vi "Compare VIs.vi"(7 "Interactive? (F)":bool, 8 "error in (no error)":errorcluster, 9 "VI Comparison Options":T1={"VI Attributes?"=TRUE, "Front Panel"=FALSE, "Front Panel Position/Size"=FALSE, "Block Diagram"=TRUE, "Block Diagram Cosmetic"=FALSE, "Block Diagram Position/Size"=FALSE}, 10 "VI Path 2":path, 11 "VI Path 1":path) -> (0 "error out":errorcluster, 3 "Different?":bool)   [LabVIEW 2016, in "SLL Scripting.lvlib"]
doc: "Compare two VIs provided their path."
uses:
  SLL Scripting.lvlib
  _Typedefs/VI Comparison Options.ctl
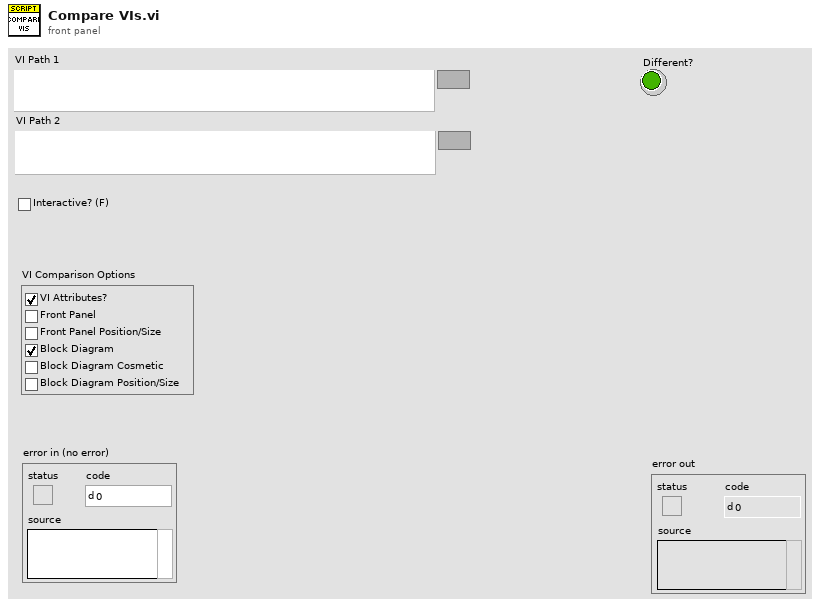
[diagram p1: front panel]
types:
  T1 = typedef "SLL Scripting.lvlib/VI Comparison Options.ctl" = cluster{"VI Attributes?":bool, "Front Panel":bool, "Front Panel Position/Size":bool, "Block Diagram":bool, "Block Diagram Cosmetic":bool, "Block Diagram Position/Size":bool}
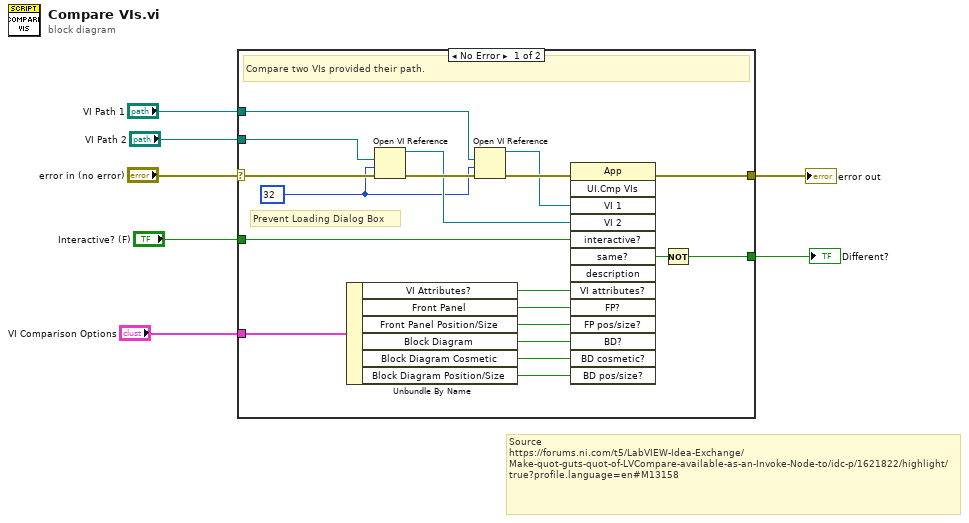
[diagram p0: block diagram]
diagram:
  # "Source\nhttps://forums.ni.com/t5/LabVIEW-Idea-Exchange/Make-quot-guts-quot-of-LVCompare-available-as-an-Invoke-Node-to/idc-p/1621822/highlight/true?profile.language=en#M13158"
  n1 = case shown="No Error" "error in (no error)" {
    selector: "error in (no error)" -> [w17 w27]
    tunnel: [w9 _] -> w7
    tunnel: "Interactive? (F)" -> [w25 _]
    tunnel: "VI Comparison Options" -> [w24 _]
    tunnel: [w16 w27] -> w3
    tunnel: "VI Path 1" -> [w13 _]
    tunnel: "VI Path 2" -> [w12 _]
    frame No Error {
      w8 = 32 ("options")
      # "Prevent Loading Dialog Box"
      # "Compare two VIs provided their path."
      n2 = Unbundle By Name(w24) -> ("VI Attributes?"=w23:bool, "Front Panel"=w22:bool, "Front Panel Position/Size"=w21:bool, "Block Diagram"=w20:bool, "Block Diagram Cosmetic"=w19:bool, "Block Diagram Position/Size"=w18:bool)
      n3 = Open VI Reference(vi path=w12, options=w8, error in (no error)=w17) -> (vi reference=w10:refnum<vi>, error out=w15:errorcluster)  [unwired: 3 in]
      n4 = Open VI Reference(vi path=w13, options=w8, error in (no error)=w15) -> (vi reference=w11:refnum<vi>, error out=w14:errorcluster)  [unwired: 3 in]
      n5 = invoke class="App" method="UI.Cmp VIs"(error in=w14, "VI 1"=w11, "VI 2"=w10, "interactive?"=w25, "VI attributes?"=w23, "FP?"=w22, "FP pos/size?"=w21, "BD?"=w20, "BD cosmetic?"=w19, "BD pos/size?"=w18) -> (error out=w16:errorcluster, "same?"=w26:bool)  [unwired: 4 in, 12 out]
      n6 = Not(x=w26) -> (.not. x?=w9:bool)
    }
    frame Error {
    }
  }
  "Different?" <- w7
  "error out" <- w3
